vi "CMWtestsubscribe.vi"(8 "error in (no error)":errorcluster, 11 "URL":string="VAC.VGHA_41677/PR") -> (0 "error out":errorcluster, 2 "CMWdbl":string, 3 "Numeric":sgl)   [LabVIEW 2014]
uses:
  <userlib>/_RADE/RIO/CMW/classes/CMWSubscribe/openCMWSubscribe.vi
  <userlib>/_RADE/RIO/CMW/classes/CMWSubscribe/CMWSubscribe.vi
  <userlib>/_RADE/RIO/CMW/classes/CMWSubscribe/CMWSubscribe.lvclass
panel:
  out "Data":variant
  out "Loop":i32
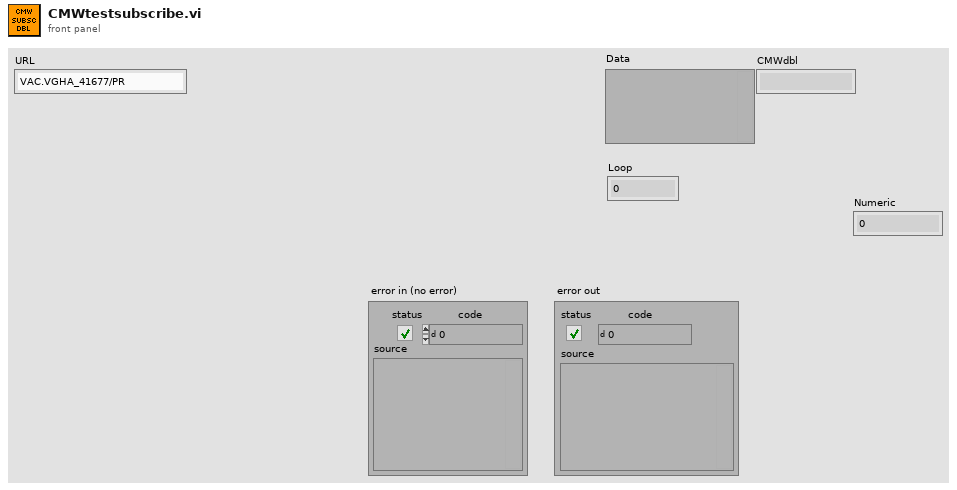
[diagram p1: front panel]
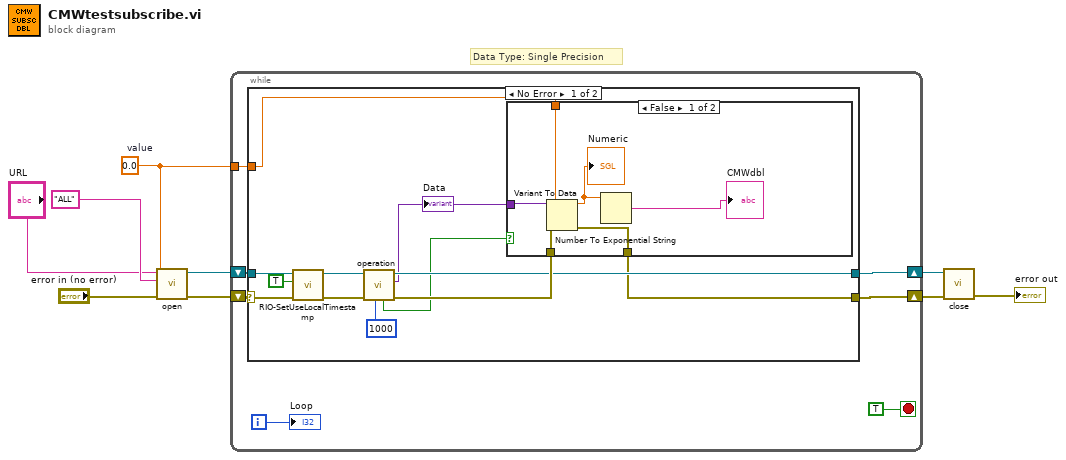
[diagram p0: block diagram]
diagram:
  w3 = sgl 0.0  # value
  # "Data Type: Single Precision"
  n1 = call-poly <userlib>:"open.vi"("error in (no error)"="error in (no error)", "Data type"=w3, "Cycle"="ALL", "URL"="URL") -> ("error out"=w7:errorcluster, "Object out"=w6:refnum<class "CMWSubscribe.lvclass">)  [unwired: 6 in]
  n2 = while {
    shift-right: [w14] -> w5
    shift-left: w7 -> [w16]
    shift-right: [w12] -> w4
    shift-left: w6 -> [w13]
    tunnel: w3 -> [w11]
    i -> [w15]
    stop <- TRUE stop-if-true
    n3 = case shown="No Error" w16 {
      selector: w16 -> [w22 w37]
      tunnel: [w26 w37] -> w14
      tunnel: w13 -> [w20 w36]
      tunnel: [w27 w36] -> w12
      tunnel: w11 -> [w25 _]
      frame No Error {
        n4 = call-dynamic "RIO-SetUseLocalTimestamp.vi"("error in (no error)"=w22, "Use Local Timestamp?"=TRUE, "CMWBase in"=w20) -> ("error out"=w21:errorcluster, "CMWBase out"=w19:refnum<class "CMWSubscribe.lvclass">)  [unwired: 7 in]
        n5 = call-poly <userlib>:"operation.vi"("Timeout (10000 ms)"=1000, "error in (no error)"=w21, "Object in"=w19) -> ("error out"=w28:errorcluster, "Data"=w17:variant, "Object out"=w27:refnum<class "CMWSubscribe.lvclass">, "Timeout?"=w23:bool)  [unwired: 4 in, 1 out]
        "Data" <- w17
        n6 = case shown="False" w23 {
          tunnel: w28 -> [w34 w35]
          tunnel: [w31 w35] -> w26
          tunnel: w17 -> [w33 _]
          tunnel: w25 -> [w32 _]
          frame False {
            n7 = Variant To Data(error in=w34, type=w32, Variant=w33) -> (data=w30:sgl, error out=w31:errorcluster)
            "Numeric" <- w30
            n8 = Number To Exponential String(number=w30) -> (E-format string=→"CMWdbl":string)  [unwired: 3 in]
          }
          frame True {
          }
        }
      }
      frame Error {
      }
    }
    "Loop" <- w15
  }
  n9 = call-dynamic "close.vi"("error in (no error)"=w5, "Object in"=w4) -> ("error out"=→"error out":errorcluster)  [unwired: 9 in]
